vi "controls_indicators.vi"() -> ()   [LabVIEW 2014]
panel:
  out "error out":errorcluster
  in  "error in (no error)":errorcluster
  out "Time Stamp 2":timestamp
  in  "Time Stamp":timestamp
  out "Enum Indicator":enum16{""}(ring)
  in  "Enum Control":enum16{""}(ring)
  out "String Indicator":string
  in  "String Control":string
  out "Boolean Indicator":bool
  in  "Boolean Control":bool
  out "Meter":dbl(knob) scale=0.0..10.0
  in  "Slide":dbl(slide) scale=0.0..10.0
  out "Thermometer":dbl(slide) scale=0.0..100.0
  in  "Knob":dbl(knob) scale=0.0..10.0
  out "Numeric Indicator":dbl
  in  "Numeric Control":dbl
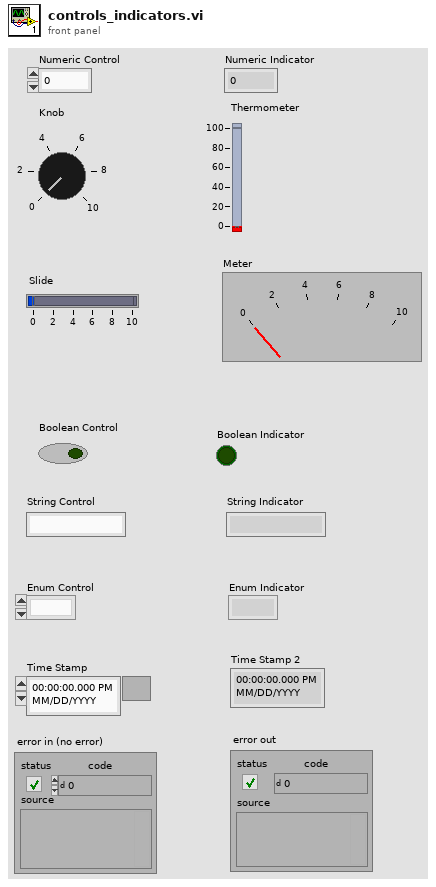
[diagram p1: front panel]
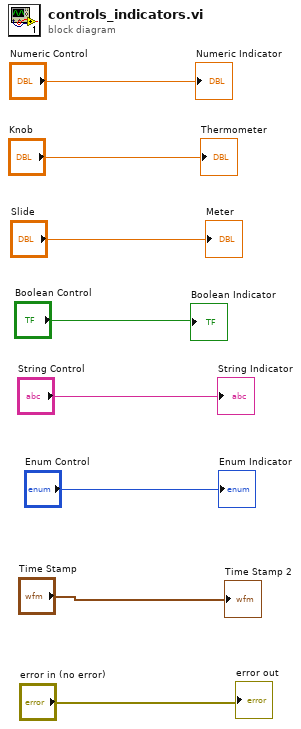
[diagram p0: block diagram]
diagram:
  "Numeric Indicator" <- "Numeric Control"
  "Thermometer" <- "Knob"
  "Meter" <- "Slide"
  "Boolean Indicator" <- "Boolean Control"
  "String Indicator" <- "String Control"
  "Enum Indicator" <- "Enum Control"
  "Time Stamp 2" <- "Time Stamp"
  "error out" <- "error in (no error)"
